vi "CTR Start.vi"(8 "error in (no error)":errorcluster, 11 "NI Counter IO in":refnum<class "NI Counter IO.lvclass">) -> (0 "error out":errorcluster, 3 "NI Counter IO out":refnum<class "NI Counter IO.lvclass">)   [LabVIEW 2020, in "NI DAQmx.lvlib" / "NI Counter IO.lvclass"]
uses:
  NI Counter IO.lvclass
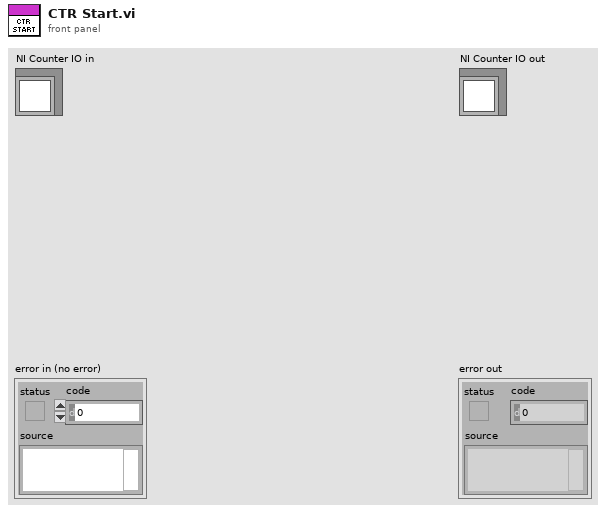
[diagram p1: front panel]
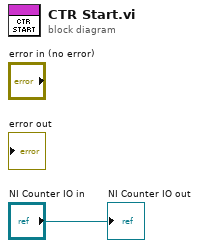
[diagram p0: block diagram]
diagram:
  "NI Counter IO out" <- "NI Counter IO in"
